vi "tearDown.vi"(8 "error in (no error)":errorcluster, 11 "reference in":refnum<class "testcase-csm-file-logger.lvclass">) -> (0 "error out":errorcluster, 3 "reference out":refnum<class "testcase-csm-file-logger.lvclass">)   [LabVIEW 2017, in "testcase-csm-file-logger.lvclass"]
doc: "tearDown runs after the test method has completed. Use this method to clean up any operations or references that were opened by setUp or the test method. Unit tests should be independent of other unit tests so this VI should ensure that the next test can run in a 'clean' test environment."
uses:
  testcase-csm-file-logger.lvclass
  testcase-csm-file-logger.lvclass/testcase-csm-file-logger.ctl
  user.lib/_NEVSTOP/Communicable State Machine(CSM)/_Support/Priority Queue/Priority Queue.lvclass/Priority Queue.ctl
  user.lib/_NEVSTOP/Communicable State Machine(CSM)/_Support/Process/CSMP-Sync Call.vi
  user.lib/_NEVSTOP/Communicable State Machine(CSM)/Utility/uuid.vi
  user.lib/_NEVSTOP/Communicable State Machine(CSM)/Utility/Build Error Cluster.vi
  user.lib/_NEVSTOP/Communicable State Machine(CSM)/Utility/Trim Both Whitespace.vi
  user.lib/_NEVSTOP/Communicable State Machine(CSM)/_Support/CSMQ/_CSMObj-Message Check.vi
  user.lib/_NEVSTOP/Communicable State Machine(CSM)/_Support/CSMQ/_CSMObj-Enqueue Cross-Module Message.vi
  user.lib/_NEVSTOP/Communicable State Machine(CSM)/_Support/CSMQ/_CSMOFGV Get.vi
  user.lib/_NEVSTOP/Communicable State Machine(CSM)/_Support/Priority Queue/Enqueue Element.vi
  user.lib/_NEVSTOP/Communicable State Machine(CSM)/_Support/Error/CSM No Target Error.vi
  user.lib/_NEVSTOP/Communicable State Machine(CSM)/_Support/CSMQ/_CSMOFGV.vi
  user.lib/_NEVSTOP/Communicable State Machine(CSM)/_Support/Error/CSM Not Allowed Message.vi
  user.lib/_NEVSTOP/Communicable State Machine(CSM)/_Support/Error/CSM Target Error.vi
  user.lib/_NEVSTOP/Communicable State Machine(CSM)/_Support/Error/CSM Unhandled State Error.vi
  user.lib/_NEVSTOP/Communicable State Machine(CSM)/_Support/Error/CSM Target Timeout Error.vi
  user.lib/_NEVSTOP/Communicable State Machine(CSM)/Communicable State Machine.lvlib
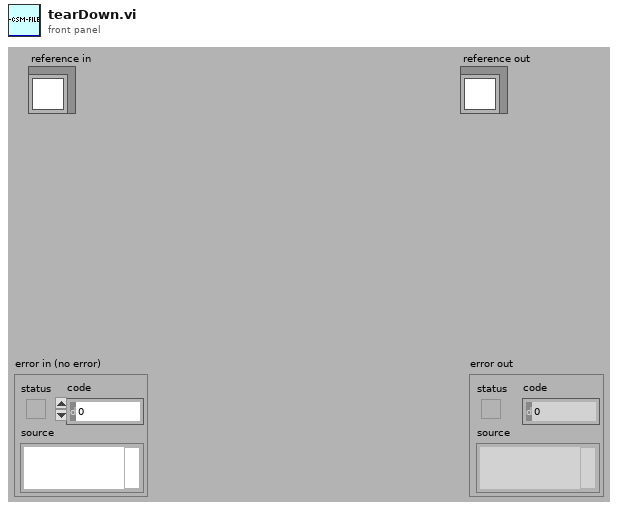
[diagram p1: front panel]
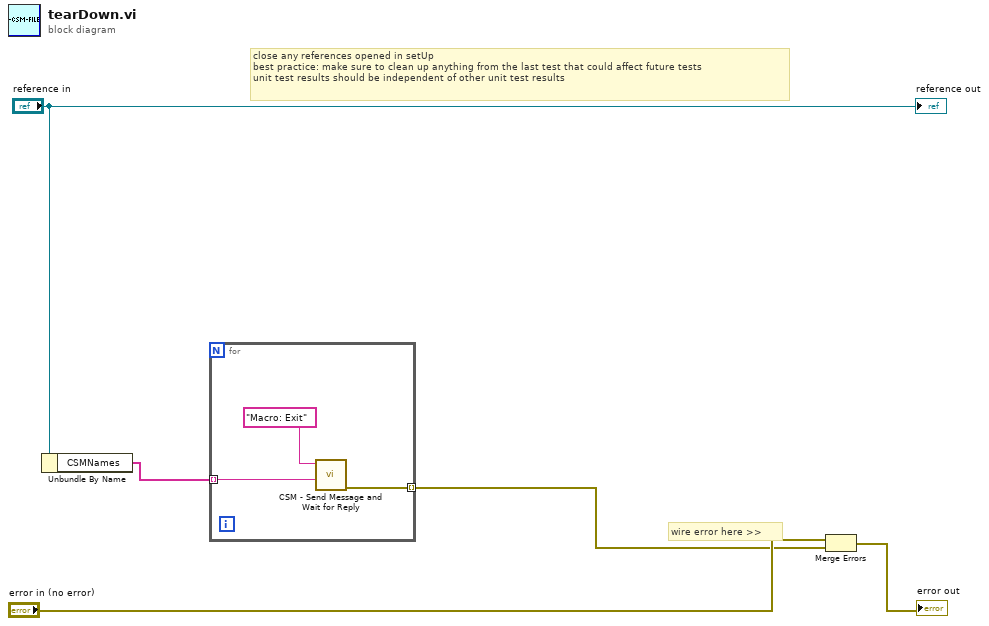
[diagram p0: block diagram]
diagram:
  # "wire error here >>"
  # "close any references opened in setUp\nbest practice: make sure to clean up anything from the last test that could affect future tests\nunit test results should be independent of other unit test results"
  n1 = Unbundle By Name("reference in") -> ("CSMNames"=w2:string[])
  n2 = for {
    tunnel: w2 -> [w7] mode=indexing
    tunnel: [w6] -> w1 mode=indexing
    n3 = call "CSM - Send Message and Wait for Reply.vi"("Target Module"=w7, "State"="Macro: Exit") -> ("error out"=w6:errorcluster)  [unwired: 7 in, 2 out]
  }
  n4 = Merge Errors("error in (no error)", w1) -> (→"error out":errorcluster)
  "reference out" <- "reference in"
